vi "Update Queue Nested.vi"(10 "Queue Nested":map{string, refnum<data-value>}(c390), 11 "jettl Event Actor in":refnum<class "jettl Event Actor.lvclass">) -> (3 "jettl Event Actor out":refnum<class "jettl Event Actor.lvclass">)   [LabVIEW 2021, in "jettl.lvlib" / "jettl Event Actor.lvclass"]
uses:
  jettl Event Actor.lvclass
  jettl Event Actor.lvclass/jettl Event Actor.ctl
  Actor/Msg/Msg.lvclass
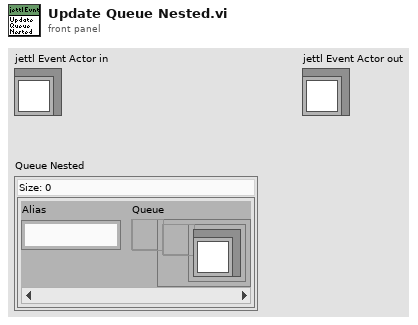
[diagram p1: front panel]
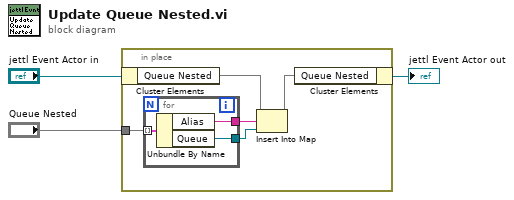
[diagram p0: block diagram]
diagram:
  n1 = in-place {
    in-place-border: "Queue Nested" -> [w6]
    n2 = in-place-cluster #1("jettl Event Actor in") -> ("Queue Nested"=w8:map{string, refnum<data-value>})
    n3 = for {
      tunnel: w6 -> [w11] mode=indexing
      tunnel: [w10] -> w5
      tunnel: [w9] -> w4
      n4 = Unbundle By Name(w11) -> ("Alias"=w10:string, "Queue"=w9:refnum<data-value>)
    }
    n5 = Insert Into Map(map in=w8, key=w5, value=w4) -> (map out=w7:map{string, refnum<data-value>})  [unwired: 2 out]
    n6 = in-place-cluster #1("Queue Nested"=w7) -> (→"jettl Event Actor out":refnum<class "jettl Event Actor.lvclass">)
  }
